vi "DelayWriteInfo.vi"(0 "Delay position input (ps)":dbl format="%#_30g") -> ()   [LabVIEW 2013]
uses:
  <vilib>/Utility/file.llb/Read From Spreadsheet File (DBL).vi
  <vilib>/Utility/file.llb/Write To Spreadsheet File (DBL).vi
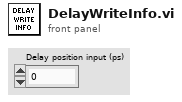
[diagram p1: front panel]
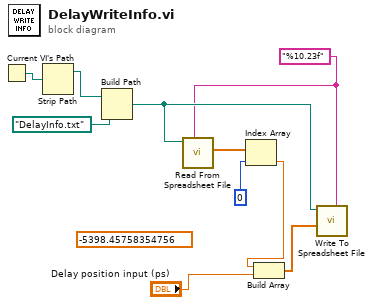
[diagram p0: block diagram]
diagram:
  (unwired) -5398.45758354756
  w4 = "%10.23f"
  n1 = Current VI's Path() -> (path=w9:path)
  n2 = Strip Path(path=w9) -> (stripped path=w8:path)  [unwired: 1 out]
  n3 = Build Path(base path=w8, name or relative path=path "DelayInfo.txt") -> (appended path=w5:path)
  n4 = call-poly <vilib>:"Read From Spreadsheet File.vi"("format (%.3f)"=w4, "file path (dialog if empty)"=w5) -> ("first row"=w3:dbl[])  [unwired: 5 in, 4 out]
  n5 = Index Array(array=w3, index=0) -> (element=w1:dbl)
  n6 = Build Array(w1, "Delay position input (ps)") -> (w7:dbl[])
  n7 = call-poly <vilib>:"Write To Spreadsheet File.vi"("format (%.3f)"=w4, "1D data"=w7, "file path (dialog if empty)"=w5) -> ()  [unwired: 5 in, 1 out]
